vi "Get Text Rect with Pad.vi"(2 "Text":string, 3 "Origin(0,0)":cluster{"horizontal":i16, "vertical":i16}, 4 "Font":T2) -> (0 "Width":i16, 1 "Rect":T1)   [LabVIEW 2017]
doc: "Measures the rectangle needed to draw Text in the given font, then pads the width by 10 percent to correct for measurement inaccuracy."
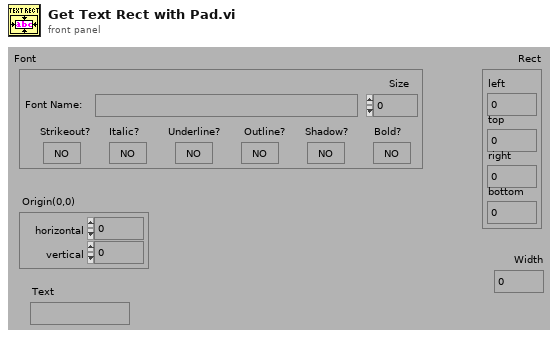
[diagram p1: front panel]
types:
  T1 = cluster{"left":i16, "top":i16, "right":i16, "bottom":i16}
  T2 = cluster{"Font Name:":string, "Size":i16, "Strikeout?":bool, "Italic?":bool, "Underline?":bool, "Outline?":bool, "Shadow?":bool, "Bold?":bool}
  T3 = enum16{"User-specified Font", "Application Font", "System Font", "Dialog Font"}
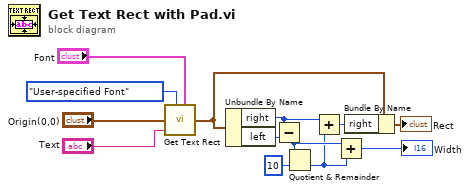
[diagram p0: block diagram]
diagram:
  n1 = call <vilib>:"Get Text Rect.vi"("desired font(Application)"=T3."User-specified Font" ("desired font(application)"), "origin(0,0)"="Origin(0,0)", "text"="Text", "[user-specified font]"="Font") -> ("rect"=w9:T1)  [unwired: 5 in]
  n2 = Unbundle By Name(w9) -> ("right"=w5:i16, "left"=w6:i16)
  n3 = Subtract(x=w5, y=w6) -> (x-y=w3:i16)
  n4 = Quotient & Remainder(x=w3, y=i16 10) -> (floor(x/y)=w2:i16)  [unwired: 1 out]
  n5 = Add(x=w5, y=w2) -> (x+y=w4:i16)
  n6 = Add(x=w3, y=w2) -> (x+y=→"Width":i16)
  n7 = Bundle By Name(cluster=w9, "right"=w4) -> (→"Rect":T1)
